vi "Set_State_BB.vi"   [LabVIEW 2012]
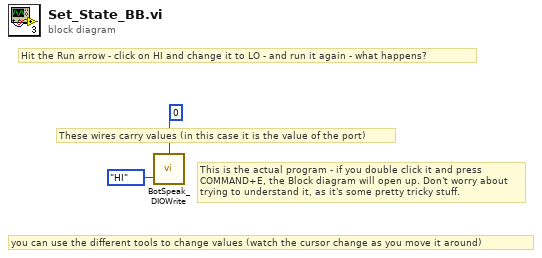
[diagram p0: block diagram]
diagram:
  # "This is the actual program - if you double click it and press COMMAND+E, the Block diagram will open up. Don't worry about trying to understand it, as it's some pretty tricky stuff."
  # "These wires carry values (in this case it is the value of the port)"
  # "you can use the different tools to change values (watch the cursor change as you move it around)"
  # "Hit the Run arrow - click on HI and change it to LO - and run it again - what happens?"
  n1 = call <userlib>:"BotSpeak_DIOWrite.vi"("State"=enum32{"LO", "HI"}."HI", "DIO Line"=u32 0) -> ()  [unwired: 1 in, 2 out]
